vi "rtPosition.vi"(8 "Calib High (in)":sgl, 9 "Calib Low (in)":sgl, 11 "Measure (mA)":dbl) -> (2 "Block Position (ft)":dbl, 3 "Block Position (in)":dbl)   [LabVIEW 2019]
panel:
  # "Block Position"
  # "Banner Time of Flight Laser Distance Meter"
  # "Calibration Data"
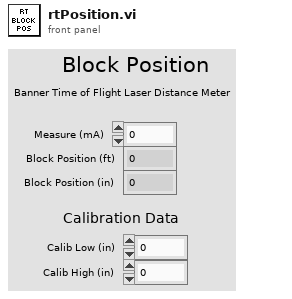
[diagram p1: front panel]
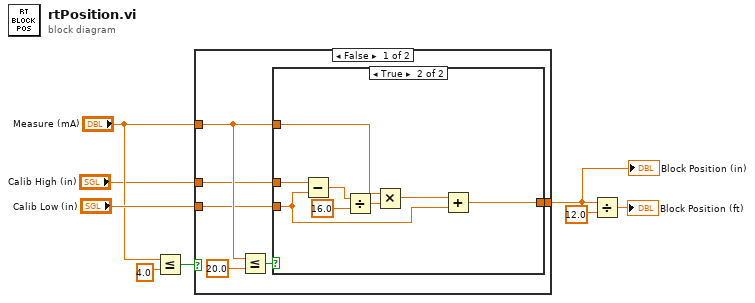
[diagram p0: block diagram]
diagram:
  n1 = Less Or Equal?(x="Measure (mA)", y=4.0) -> (x <= y?=w8:bool)
  n2 = case shown="False" w8 {
    tunnel: "Calib Low (in)" -> [w10 w24]
    tunnel: [w9 w24] -> w1
    tunnel: "Measure (mA)" -> [w12 _]
    tunnel: "Calib High (in)" -> [w11 _]
    frame False {
      n3 = Less Or Equal?(x=w12, y=20.0) -> (x <= y?=w14:bool)
      n4 = case shown="True" w14 {
        tunnel: w12 -> [_ w19]
        tunnel: w11 -> [w15 w23]
        tunnel: w10 -> [_ w17]
        tunnel: [w15 w16] -> w9
        frame False {
        }
        frame True {
          n5 = Subtract(x=w23, y=w17) -> (x-y=w22:sgl)
          n6 = Divide(x=w22, y=sgl 16.0) -> (x/y=w20:sgl)
          n7 = Multiply(x=w19, y=w20) -> (x*y=w18:dbl)
          n8 = Add(x=w18, y=w17) -> (x+y=w16:dbl)
        }
      }
    }
    frame True {
    }
  }
  "Block Position (in)" <- w1
  n9 = Divide(x=w1, y=sgl 12.0) -> (x/y=→"Block Position (ft)":dbl)
